vi "Device_Parse Answer to Tokens Array.vi"(8 "error in (no error)":errorcluster, 10 "Answer":string) -> (0 "error out":errorcluster, 2 "Tokens Array":string[](array[string]))   [LabVIEW 2017]
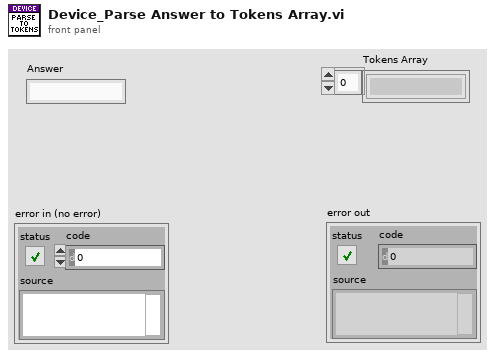
[diagram p1: front panel]
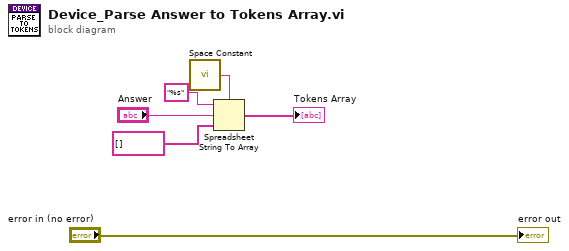
[diagram p0: block diagram]
diagram:
  n1 = call <vilib>:"Space Constant.vi"() -> ("String"=w4:string)
  n2 = Spreadsheet String To Array(delimiter (Tab)=w4, format string="%s", spreadsheet string="Answer", array type (2D Dbl)=string[] [] ("Tokens Array 2")) -> (array=→"Tokens Array":string[])
  "error out" <- "error in (no error)"
